vi "merFISH_write_injection_line_item_name.vi"(4 "Flow rate (µl/min)":i32, 5 "Select product":i32, 6 "Injection line number":i32, 7 "Buffer list":string[][](array[string]), 8 "Volume (µl)":i32, 9 "Pressure (mbar)":i32) -> (2 "Task name":string)   [LabVIEW 2015]
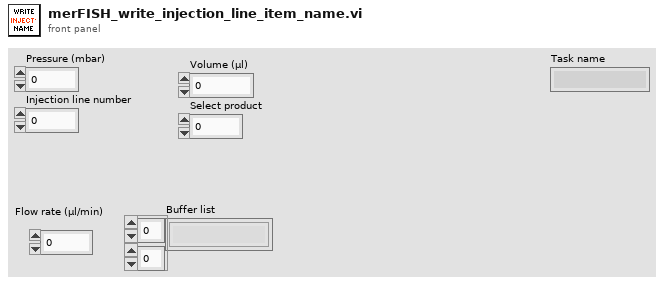
[diagram p1: front panel]
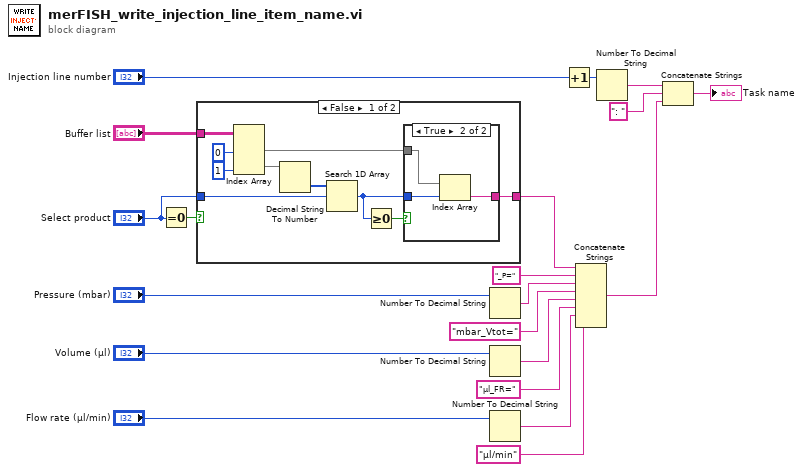
[diagram p0: block diagram]
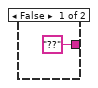
[diagram p2: hidden frame]
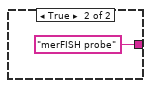
[diagram p3: hidden frame]
diagram:
  n1 = Equal To 0?(x="Select product") -> (x = 0?=w7:bool)
  n2 = case shown="False" w7 {
    tunnel: [w21 "merFISH probe" ("new element/subarray")] -> w1
    tunnel: "Buffer list" -> [w30 _]
    tunnel: "Select product" -> [w26 _]
    frame False {
      n3 = Index Array(array=w30, index (col) #1=0 ("disabled index (col)"), index (col) #2=1 ("disabled index (col)")) -> (element #1=w23:string[], element #2=w28:string[])  [unwired: 2 in]
      n4 = Decimal String To Number(string=w28) -> (number=w27:i32[])  [unwired: 2 in, 1 out]
      n5 = Search 1D Array(1D array=w27, element=w26) -> (index of element=w22:i32)  [unwired: 1 in]
      n6 = Greater Or Equal To 0?(x=w22) -> (x >= 0?=w25:bool)
      n7 = case shown="True" w25 {
        tunnel: w23 -> [_ w34]
        tunnel: w22 -> [_ w33]
        tunnel: ["??" w32] -> w21
        frame False {
        }
        frame True {
          n8 = Index Array(array=w34, index=w33) -> (element=w32:string)
        }
      }
    }
    frame True {
    }
  }
  n9 = Number To Decimal String(number="Pressure (mbar)") -> (decimal integer string=w17:string)  [unwired: 1 in]
  n10 = Number To Decimal String(number="Volume (µl)") -> (decimal integer string=w19:string)  [unwired: 1 in]
  n11 = Number To Decimal String(number="Flow rate (µl/min)") -> (decimal integer string=w4:string)  [unwired: 1 in]
  n12 = Increment(x="Injection line number") -> (x+1=w12:i32)
  n13 = Concatenate Strings(w1, "_P=" ("string"), w17, "mbar_Vtot=" ("string"), w19, "µl_FR=" ("string"), w4, "µl/min" ("string")) -> (w15:string)
  n14 = Number To Decimal String(number=w12) -> (decimal integer string=w13:string)  [unwired: 1 in]
  n15 = Concatenate Strings(w13, ": " ("string"), w15) -> (→"Task name":string)
